vi "JSON Read User Event_Algo.vi"(8 "error in (no error)":errorcluster, 10 "JSON Read":T1, 11 "Algorithm in":refnum<class "Algorithm.lvclass">) -> (0 "error out":errorcluster, 3 "Algorithm out":refnum<class "Algorithm.lvclass">)   [LabVIEW 2015]
uses:
  FrameworkOverrides/Algorithm.lvclass
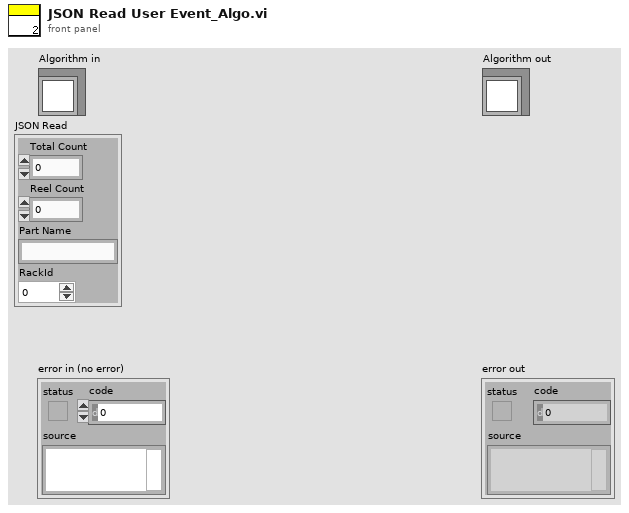
[diagram p1: front panel]
types:
  T1 = cluster{"Total Count":u64, "Reel Count":u64, "Part Name":string, "RackId":i32}
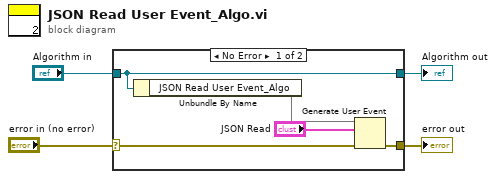
[diagram p0: block diagram]
diagram:
  n1 = case shown="No Error" "error in (no error)" {
    selector: "error in (no error)" -> [w7 w11]
    tunnel: [w6 w11] -> w3
    tunnel: [w9 w10] -> w1
    tunnel: "Algorithm in" -> [w9 w10]
    frame No Error {
      n2 = Unbundle By Name(w9) -> ("JSON Read User Event_Algo"=w8)
      n3 = Generate User Event(user event=w8, event data cluster="JSON Read", error in=w7) -> (error out=w6:errorcluster)  [unwired: 1 in, 1 out]
    }
    frame Error {
    }
  }
  "error out" <- w3
  "Algorithm out" <- w1
